vi "Switching Mechanical Actions.vi"() -> ()   [LabVIEW 2020]
panel:
  out "Switch Until Released":bool
  out "Switch When Released":bool
  out "Switch When Pressed":bool
  in  "Switch Until Released":bool
  in  "Switch When Released":bool
  in  "Switch When Pressed":bool
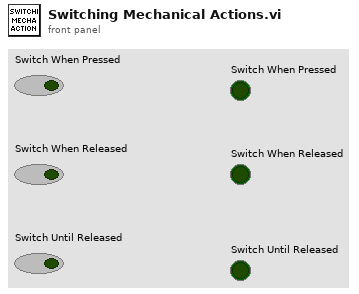
[diagram p1: front panel]
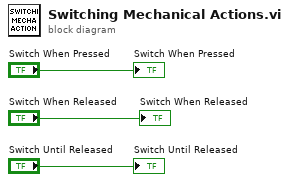
[diagram p0: block diagram]
diagram:
  "Switch When Pressed" <- "Switch When Pressed"
  "Switch When Released" <- "Switch When Released"
  "Switch Until Released" <- "Switch Until Released"
